vi "Configure RTD Type.vi"(8 "error in (no error)":errorcluster, 9 "Resistance at 0°C(100Ohm)":dbl=100.0, 10 "RTD Type":T1=enum."Pt3851" caption="RTD Type(Pt3851)", 11 "DMM Driver in":refnum<class "DMM Driver.lvclass">) -> (0 "error out":errorcluster, 1 "Success?":bool, 3 "DMM Driver out":refnum<class "DMM Driver.lvclass">)   [LabVIEW 2020, in "DMM.lvlib" / "DMM Driver.lvclass"]
doc: "Configure the RTD type used when measuring temperatures."
uses:
  DMM Driver.lvclass
  Controls/Ctl_RTDType.ctl
  DMM.lvlib
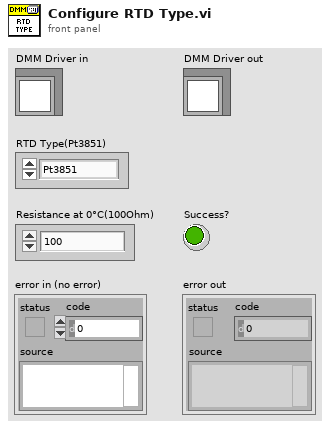
[diagram p1: front panel]
types:
  T1 = typedef "DMM.lvlib/Ctl_RTDType.ctl" = enum16{"Custom", "Pt3750", "Pt3851", "Pt3911", "Pt3916", "Pt3920", "Pt3928"}
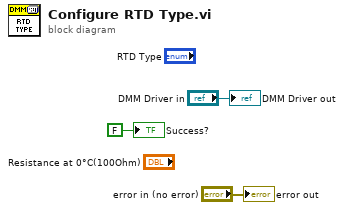
[diagram p0: block diagram]
diagram:
  "error out" <- "error in (no error)"
  "DMM Driver out" <- "DMM Driver in"
  "Success?" <- FALSE ("Success?")
